vi "Ramp to Set.vi"(8 "error in (no error)":errorcluster, 11 "Instrument.1820 in":refnum<class "Instrument.Oxford1820.lvclass">) -> (0 "error out":errorcluster, 2 "Response":string, 3 "Instrument.1820 in":refnum<class "Instrument.Oxford1820.lvclass">)   [LabVIEW 2019, in "Instrument.Oxford1820.lvclass"]
uses:
  Instrument.Oxford1820.lvclass
  Typedefs/Instrument.Oxford1820.protectedCommands-enum.ctl
  87657c41-108c-4a48-bbe5-bc3f5bda3d1d.vi/ef46835e-a967-4727-9395-1b72a8dcca00.vi
  87657c41-108c-4a48-bbe5-bc3f5bda3d1d.vi/ce9bce06-d4b6-4e9d-a627-04ae8f197ac2.vi
  <vilib>/Utility/Data Type/Get Type Information.vi
  <vilib>/JDP Science/JSONtext/JSON text to Variant.vi
  <vilib>/JDP Science/JSONtext/LVClass Serializer/JSONtext LVClass Serializer.lvclass
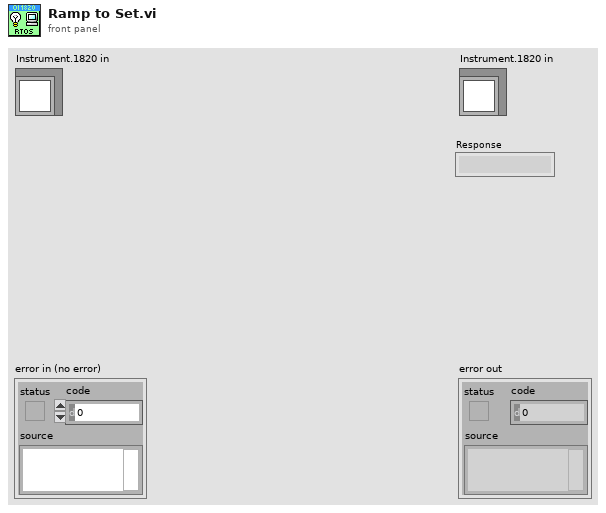
[diagram p1: front panel]
types:
  T1 = typedef "Instrument.Oxford1820.lvclass/Instrument.Oxford1820.protectedCommands-enum.ctl" = enum16{"Hold", "RampToSet", "RampToZero", "Clamp", "setTarget", "setSwitchHeat", "setLambda", "setFillMode", "setNeedleValve", "getStatus", "getTarget", "getSwitchHeat", "getPSUField", "setSequenceStatus"}
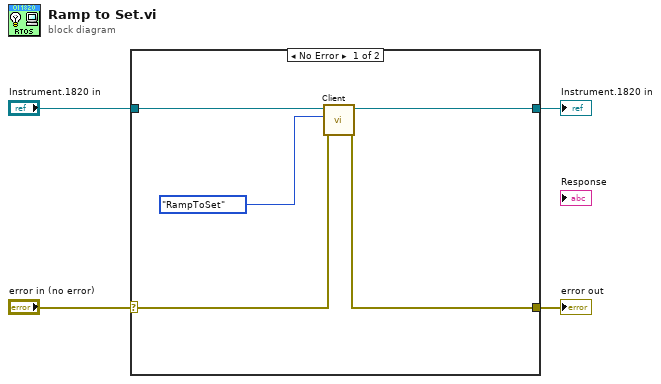
[diagram p0: block diagram]
diagram:
  n1 = case shown="No Error" "error in (no error)" {
    selector: "error in (no error)" -> [w7 w11]
    tunnel: [w5 w11] -> w3
    tunnel: [w8 w10] -> w1
    tunnel: "Instrument.1820 in" -> [w9 w10]
    frame No Error {
      n2 = call-dynamic "Client.vi"("error in (no error)"=w7, "Command in"=Instrument.Oxford1820.protectedCommands-enum."RampToSet" ("protectedCommands"), "Instrument in"=w9) -> ("error out"=w5:errorcluster, "Instrument out"=w8:refnum<class "Instrument.Oxford1820.lvclass">)  [unwired: 5 in, 2 out]
    }
    frame Error {
    }
  }
  "error out" <- w3
  "Instrument.1820 in" <- w1
